vi "3.vi"(11 "HealthAndStatusControlFIFO in":refnum<class "HealthAndStatusControlFIFO.lvclass">) -> (2 "FPGAReference":refnum<k20>, 3 "HealthAndStatusControlFIFO out":refnum<class "HealthAndStatusControlFIFO.lvclass">)   [LabVIEW 2016, in "HealthAndStatusControlFIFO.lvclass"]
uses:
  HealthAndStatusControlFIFO.lvclass
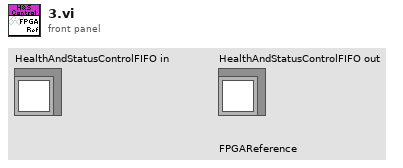
[diagram p1: front panel]
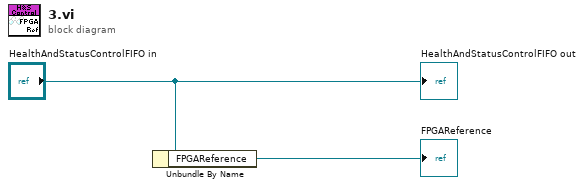
[diagram p0: block diagram]
diagram:
  n1 = Unbundle By Name("HealthAndStatusControlFIFO in") -> ("FPGAReference"=→"FPGAReference":refnum<k20>)
  "HealthAndStatusControlFIFO out" <- "HealthAndStatusControlFIFO in"
